vi "Init HTTP.vi"(8 "error in (no error)":errorcluster, 11 "System Config Server in":refnum<class "System Config Module.lvclass">) -> (0 "error out":errorcluster, 3 "System Config Server out":refnum<class "System Config Module.lvclass">)   [LabVIEW 2020, in "Volatus.lvlib" / "System Config Module.lvclass"]
uses:
  System Config Module.lvclass
  C:/dev/lv20CE/relink/lv-volatus/Volatus/Module/Module.lvclass
  Module/Module.lvclass/Module.ctl
  System Config Module.lvclass/System Config Module.ctl
  VolatusAPI/VolatusAPI.lvclass/VolatusAPI.ctl
  lv-http-server/HTTP Server/Server/Register Handler.vi
  ConfigHTTPController/ConfigHTTPController.lvclass
  C:/dev/lv20CE/relink/lv-http-server/HTTP Server/Handler/Handler.lvclass
  lv-vecto/Vecto/Vecto/Get HTTP.vi
  lv-http-server/HTTP Server/Server/Add Connection Handler.vi
  lv-http-server/HTTP Server/Server/Add Request Handler.vi
  lv-http-server/HTTP Server/Server/Add Route Handler.vi
  lv-http-server/HTTP Server/Server/Add Controller Handler.vi
  lv-http-server/HTTP Server/Server/Add Controller.vi
  lv-http-server/HTTP Server/Server/Add Response Handler.vi
  lv-http-server/HTTP Server/Server/Add Complete Handler.vi
  lv-http-server/HTTP Server/Server/Add Exception Handler.vi
  lv-http-server/HTTP Server/Connection Handler/Connection Handler.lvclass
  lv-http-server/HTTP Server/Request Handler/Request Handler.lvclass
  lv-http-server/HTTP Server/Route Handler/Route Handler.lvclass
  lv-http-server/HTTP Server/Controller Handler/Controller Handler.lvclass
  lv-http-server/HTTP Server/Controller/Controller.lvclass
  lv-http-server/HTTP Server/Response Handler/Response Handler.lvclass
  lv-http-server/HTTP Server/Complete Handler/Complete Handler.lvclass
  lv-http-server/HTTP Server/Exception Handler/Exception Handler.lvclass
  lv-http-server/HTTP Server/Handler/Handler.lvclass
  Module/Module.lvclass
  VolatusAPI/VolatusAPI.lvclass
  Nav Route/Nav Route.lvclass
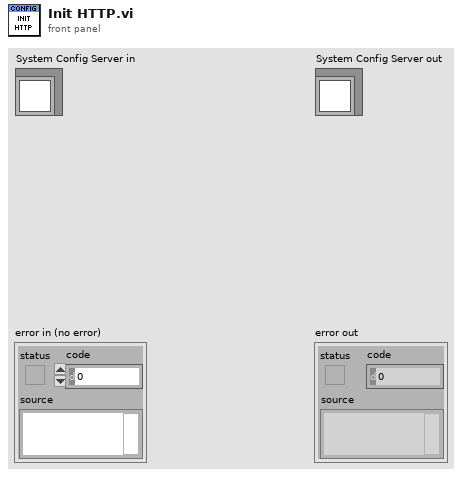
[diagram p1: front panel]
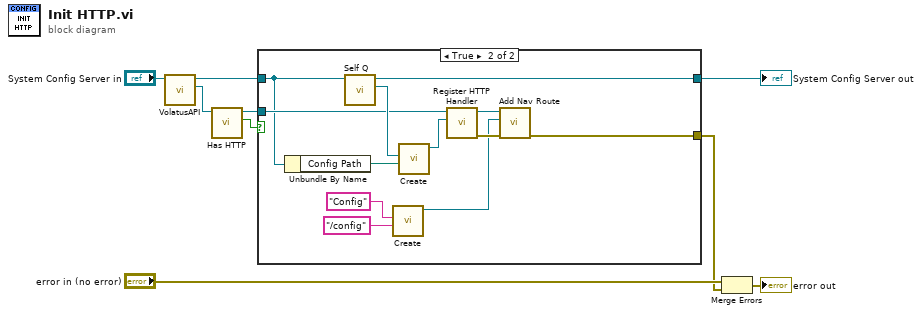
[diagram p0: block diagram]
diagram:
  n1 = call "VolatusAPI.vi"("Module in"="System Config Server in") -> ("VolatusAPI"=w6:refnum<class "VolatusAPI.lvclass">, "Module out"=w8:refnum<class "System Config Module.lvclass">)  [unwired: 9 in]
  n2 = call "Has HTTP.vi"("VolatusAPI in"=w6) -> ("Has HTTP"=w5:bool, "VolatusAPI out"=w4:refnum<class "VolatusAPI.lvclass">)  [unwired: 9 in]
  n3 = case shown="True" w5 {
    tunnel: w8 -> [w10 w18]
    tunnel: w4 -> [_ w21]
    tunnel: [w10 w19] -> w3
    tunnel: [_ w14] -> w1
    frame False {
    }
    frame True {
      n4 = Unbundle By Name(w18) -> ("Config Path"=w17:path)
      n5 = call "Self Q.vi"("Module in"=w18) -> ("Self Q"=w22:refnum<class "MessageQ.lvclass">, "Module out"=w19:refnum<class "System Config Module.lvclass">)  [unwired: 9 in]
      n6 = call "Create.vi"("Path"="/config", "Label"="Config") -> ("Nav Route out"=w11:refnum<class "Nav Route.lvclass">)  [unwired: 8 in, 1 out]
      n7 = call "Create.vi"("Config Path"=w17, "Config Module"=w22) -> ("ConfigHTTPController out"=w20:refnum<class "ConfigHTTPController.lvclass">)  [unwired: 8 in, 1 out]
      n8 = call "Register HTTP Handler.vi"("Handler"=w20, "VolatusAPI in"=w21) -> ("error out"=w15:errorcluster, "VolatusAPI out"=w16:refnum<class "VolatusAPI.lvclass">)  [unwired: 8 in]
      n9 = call "Add Nav Route.vi"("error in (no error)"=w15, "Nav Route"=w11, "VolatusAPI in"=w16) -> ("error out"=w14:errorcluster)  [unwired: 7 in, 1 out]
    }
  }
  "System Config Server out" <- w3
  n10 = Merge Errors("error in (no error)", w1) -> (→"error out":errorcluster)
